vi "Open.vi"(8 "error in (no error)":errorcluster, 11 "Endpoint in":refnum<class "Endpoint.lvclass">) -> (0 "error out":errorcluster, 3 "Endpoint out":refnum<class "Endpoint.lvclass">)   [LabVIEW 2020, in "Stream.lvlib" / "Endpoint.lvclass"]
uses:
  Endpoint.lvclass
  Endpoint.lvclass/Endpoint.ctl
  <vilib>/Utility/error.llb/Error Cluster From Error Code.vi
  <vilib>/ErrorRing/Error Ring.xnode
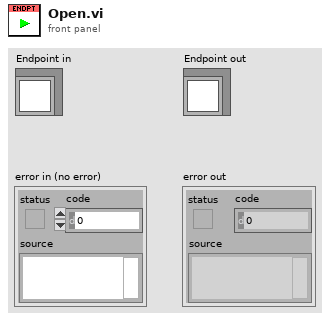
[diagram p1: front panel]
types:
  T1 = typedef "Stream.lvlib/Endpoint.lvclass/Ref Data.ctl" = cluster{"URI":refnum<class "URI.lvclass">, "State Callbacks":T2[], "Open":bool, "Mode":T3}
  T2 = typedef "Stream.lvlib/Endpoint.lvclass/State Callback.ctl" = cluster{"Owner":refnum<class>, "VI":refnum<vi>}
  T3 = typedef "Stream.lvlib/Mode.ctl" = enum16{"Raw", "Buffered", "LineTerm"}
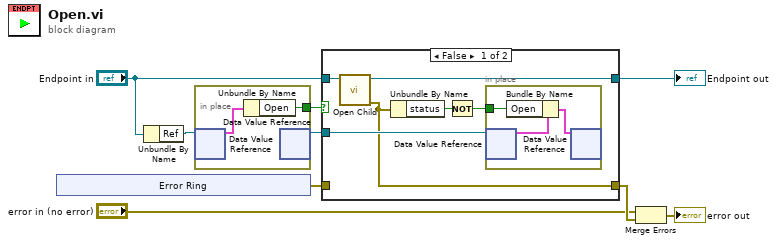
[diagram p0: block diagram]
diagram:
  n1 = xnode "Error Ring"() -> ("error out"=w4:errorcluster)
  n2 = Unbundle By Name("Endpoint in") -> ("Ref"=w9:refnum<data-value>)
  n3 = in-place {
    in-place-border: [w10] -> w8
    n4 = in-place-dvr #1(w9) -> (w11:T1)  [unwired: 1 out]
    n5 = Unbundle By Name(w11) -> ("Open"=w10:bool)
    n6 = in-place-dvr #1() -> (w6:refnum<data-value>)  [unwired: 1 in, 1 out]
  }
  n7 = case shown="False" w8 {
    tunnel: "Endpoint in" -> [w17 w22]
    tunnel: w6 -> [w15 _]
    tunnel: [w16 w22] -> w5
    tunnel: [w12 w21] -> w3
    tunnel: w4 -> [_ w21]
    frame False {
      n8 = call-dynamic "Open Child.vi"("Endpoint in"=w17) -> ("error out"=w12:errorcluster, "Endpoint out"=w16:refnum<class "Endpoint.lvclass">)  [unwired: 9 in]
      n9 = Unbundle By Name(w12) -> ("status"=w14:bool)
      n10 = Not(x=w14) -> (.not. x?=w13:bool)
      n11 = in-place {
        in-place-border: w13 -> [w18]
        n12 = in-place-dvr #2(w15) -> (w20:T1)  [unwired: 1 out]
        n13 = Bundle By Name(cluster=w20, "Open"=w18) -> (w19:T1)
        n14 = in-place-dvr #2(w19) -> ()  [unwired: 2 out]
      }
    }
    frame True {
    }
  }
  "Endpoint out" <- w5
  n15 = Merge Errors("error in (no error)", w3) -> (→"error out":errorcluster)
